vi "Load Plugin Management.vi"(11 "CIFPluginManager in":refnum<class "CIFPluginManager.lvclass">) -> (0 "error out":errorcluster)   [LabVIEW 2021, in "CIFPluginManager.lvclass"]
uses:
  CIFPluginManager.lvclass
  CIFPluginManager.lvclass/CIFPluginManager.ctl
  gRPC/CIF_Manager_server/RPC Service/Manager/Manager.lvclass
  C:/Program Files/National Instruments/LabVIEW 2021/vi.lib/gRPC/LabVIEW gRPC Servicer/ServiceBase/ServiceBase.lvclass
  gRPC/CIF_Manager_server/RPC Service/Manager/Manager.lvclass/Manager.ctl
  CIFCore/Common/Typedef/Errors.ctl
  <vilib>/Utility/miscctls.llb/LVMapReplaceAction.ctl
  <vilib>/CIF Foundation/CIF Utilities/Errors/Append Error Location.vi
  <vilib>/CIF Foundation/CIF Utilities/Time/System Time/LabVIEW Time to TAI Time.vi
  <vilib>/string/Create NI GUID.vi
  CIFUtilities/CIFLogs/CIFLogs.lvlib
  CIFCore/Common/CIFCoreCommon.lvlib
  CIFCore/Grpc/CIFCoreWrapper/CIFCoreWrapper.lvlib
  <vilib>/CIF Foundation/CIF Utilities/Time/Time_CIF_U.lvlib
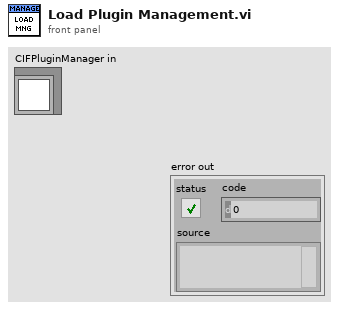
[diagram p1: front panel]
types:
  T1 = typedef "CIF_Manager_server.lvlib/Manager.lvclass/Server gRPC UEs.ctl" = cluster{"Manager LoadPlugin gRPC UE":refnum<user-event>, "Manager RegisterPlugin gRPC UE":refnum<user-event>, "Manager UnregisterPlugin gRPC UE":refnum<user-event>, "Manager QueryPluginTypes gRPC UE":refnum<user-event>, "Manager AbortPlugin gRPC UE":refnum<user-event>, "Manager UnloadAllPlugins gRPC UE":refnum<user-event>, "Manager Destroy gRPC UE":refnum<user-event>, "Manager Ping gRPC UE":refnum<user-event>, "Manager QueryErrors gRPC UE":refnum<user-event>, "Manager QueryConfig gRPC UE":refnum<user-event>, "Manager QueryInfo gRPC UE":refnum<user-event>, "Manager ResetErrorIndex gRPC UE":refnum<user-event>, "Manager ResetConfigIndex gRPC UE":refnum<user-event>, "Manager ResetInfoIndex gRPC UE":refnum<user-event>, "Manager QueryPluginInfo gRPC UE":refnum<user-event>, "Manager QueryPlugin gRPC UE":refnum<user-event>, "Manager QuerySystemStatus gRPC UE":refnum<user-event>, "Manager UpdateClock gRPC UE":refnum<user-event>, "Manager CreateOrch gRPC UE":refnum<user-event>, "Manager QueryClockStatus gRPC UE":refnum<user-event>, "Manager QueryAllChannels gRPC UE":refnum<user-event>}
  T2 = typedef "CIFCoreCommon.lvlib/Errors.ctl" = enum16{"Invalid Clock ID", "Long Sleep", "gRPC Server Not Found", "Config Parse", "Timestamp Wrap", "Delayed Execution", "Duplicate Channel", "Missing Channel", "Incorrect Type", "Flatten Error", "Unflatten Data", "Unique Name", "Plugin Not Found", "Plugin Type Not Found", "Plugin Version Not Found", "Manager Not Found", "Numerical Issue", "Time Jump", "Clock ID Match", "Channel Length", "Plugin Connection", "gRPC Server Connection", "PPL Name Match", "Build", "Config Log Parse", "Plugin Load", "UI Subpanel Load", "Python Name", "Invalid Name", "Unable to Change Ch Buffer"}
  T3 = typedef "LVMapReplaceAction.ctl" = enum32{"Modify Entry only if found", "Add or Modify Entry", "Delete Entry"}
  T4 = typedef "CIFPluginManager.lvclass/Plugin Management Data Map.ctl" = map{string, T5}
  T5 = typedef "CIFPluginManager.lvclass/Plugin Management Data.ctl" = cluster{"vi reference":refnum<vi>, "gRPC ID":T6, "Plugin Type":string, "Unique Name":string, "gRPC Port":i32, "Version":T7, "Load Timestamp":i64, "Unload Timestamp":i64, "Unloading":bool, "Ready for removal":bool, "status":T8}
  T6 = typedef "grpc-lvsupport-release.lvlib/grpcId.ctl" = u64
  T7 = typedef "CIFCoreCommon.lvlib/Version.ctl" = cluster{"Major":i32, "Minor":i32, "Fix":i32, "Build":i32}
  T8 = typedef "CIF_Manager_server.lvlib/cif_plugincore_StatusData.ctl" = cluster{"state":T9, "timing_statistics":T10, "fifo_statistics":T12, "error":T13, "monitor_doubles":T14, "monitor_u64s":T15, "monitor_i64s":T16}
  T9 = typedef "CIF_Manager_server.lvlib/cif_plugincore_StatusData_State.ctl" = enum32{"NULL", "CREATING", "LISTENING", "RUNNING", "CLEANINGUP", "DESTROYING"}
  T10 = typedef "CIF_Manager_server.lvlib/cif_plugincore_TimingStatistics.ctl" = cluster{"period":T11, "wake_error":T11, "execute":T11, "housekeep":T11, "idle":T11, "cleanup":T11, "custom_1":T11, "custom_2":T11}
  T11 = typedef "CIF_Manager_server.lvlib/cif_common_TimingStats.ctl" = cluster{"max":i64, "min":i64, "avg":dbl}
  T12 = typedef "CIF_Manager_server.lvlib/cif_plugincore_FifoStatistics.ctl" = cluster{"from_t0":T11, "from_previous_plugin":T11, "output_error":T11}
  T13 = typedef "CIF_Manager_server.lvlib/cif_plugincore_Error.ctl" = cluster{"status":bool, "code":i32}
  T14 = typedef "CIF_Manager_server.lvlib/cif_plugincore_MonitorDoubles.ctl" = cluster{"double_1":dbl, "double_2":dbl, "double_3":dbl, "double_4":dbl}
  T15 = typedef "CIF_Manager_server.lvlib/cif_plugincore_MonitorU64.ctl" = cluster{"u64_1":u64, "u64_2":u64, "u64_3":u64, "u64_4":u64}
  T16 = typedef "CIF_Manager_server.lvlib/cif_plugincore_MonitorI64.ctl" = cluster{"i64_1":i64, "i64_2":i64, "i64_3":i64, "i64_4":i64}
  T17 = typedef "CIF_Manager_server.lvlib/cif_manager_PluginConfig.ctl" = cluster{"plugin_type":string, "plugin_name":string, "version":string}
  T18 = typedef "CIFPluginManager.lvclass/Discovered Plugin.ctl" = cluster{"Filename":string, "Plugin Type":string, "Qualified name":string, "Version":T7, "Plugin Metadata":T19}
  T19 = typedef "CIFPluginManager.lvclass/Plugin Metadata.ctl" = cluster{"Description":string, "History":string, "Author":string}
  T20 = typedef "CIF_Manager_client.lvlib/cif_common_Status.ctl" = cluster{"code":i32, "message":string}
  T21 = typedef "CIF_Manager_server.lvlib/cif_manager_PluginName.ctl" = cluster{"plugin_name":string}
  T22 = typedef "Plugin Management Data Map.ctl" = map{string, T5}
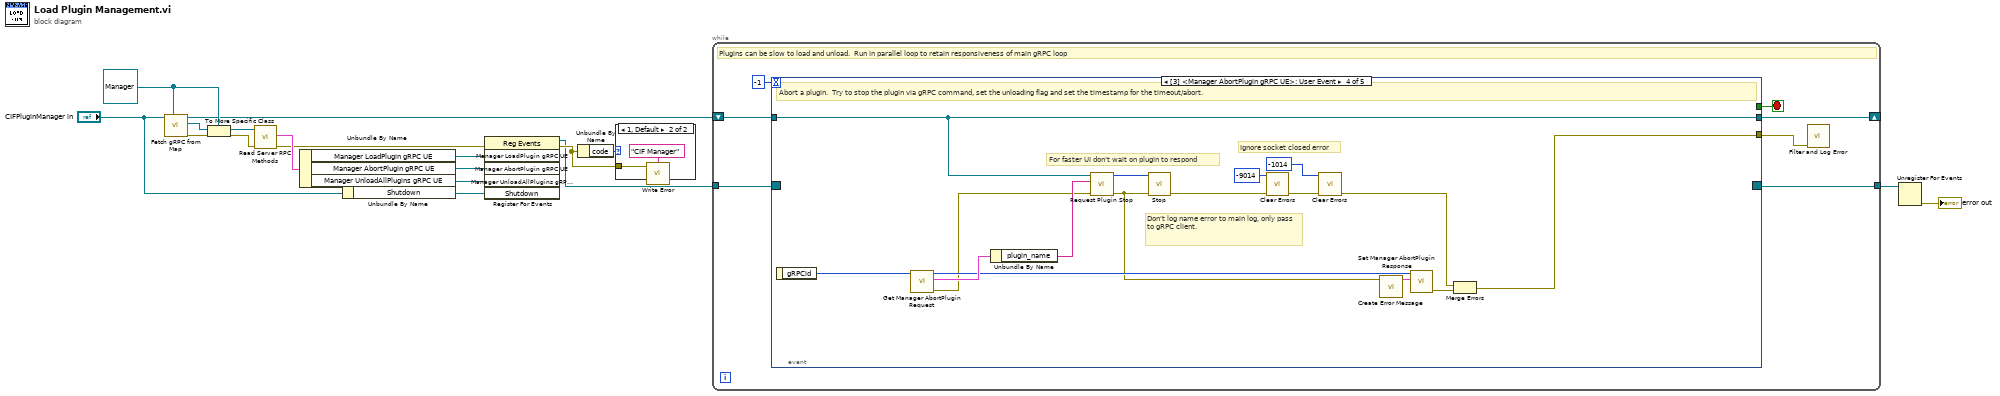
[diagram p0: block diagram]
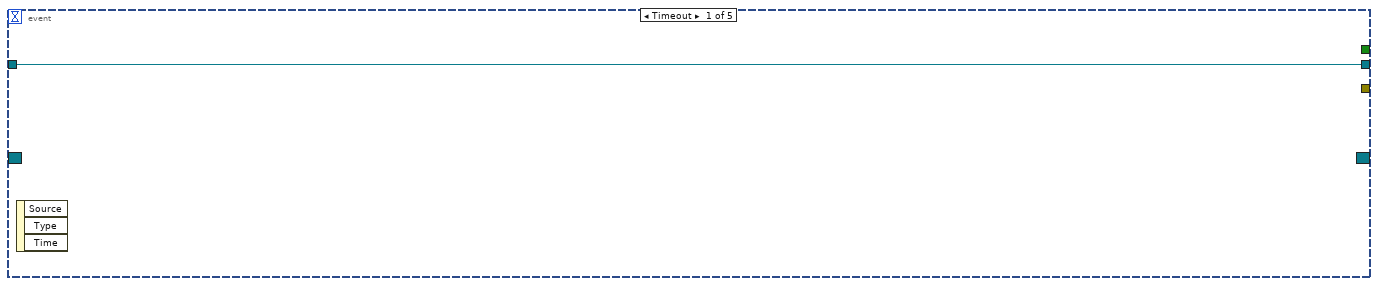
[diagram p3: hidden frame]
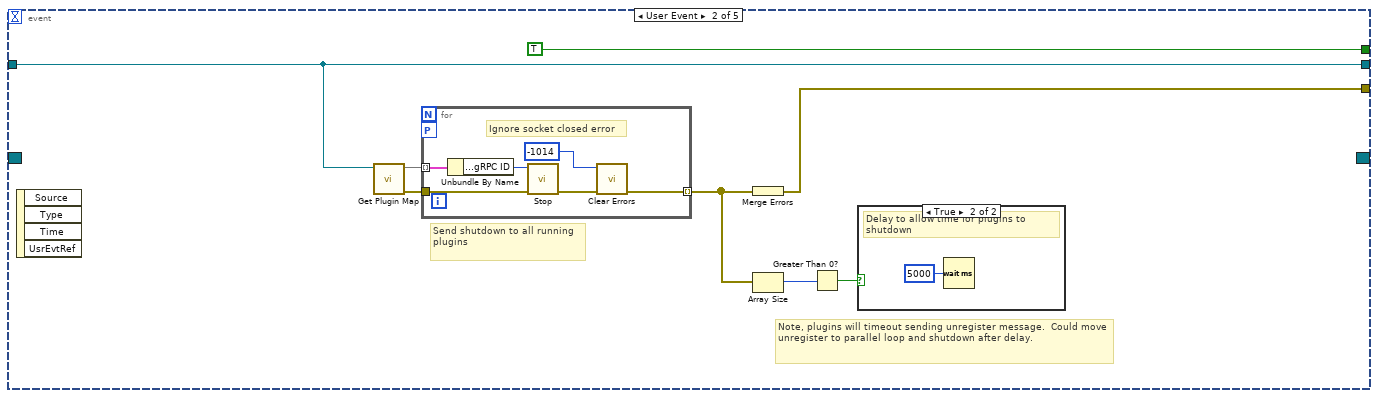
[diagram p4: hidden frame]
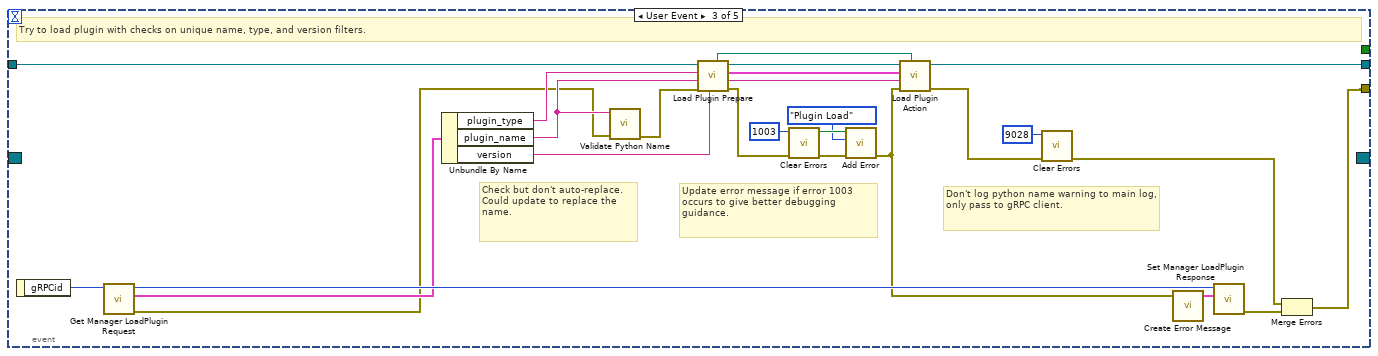
[diagram p6: hidden frame]
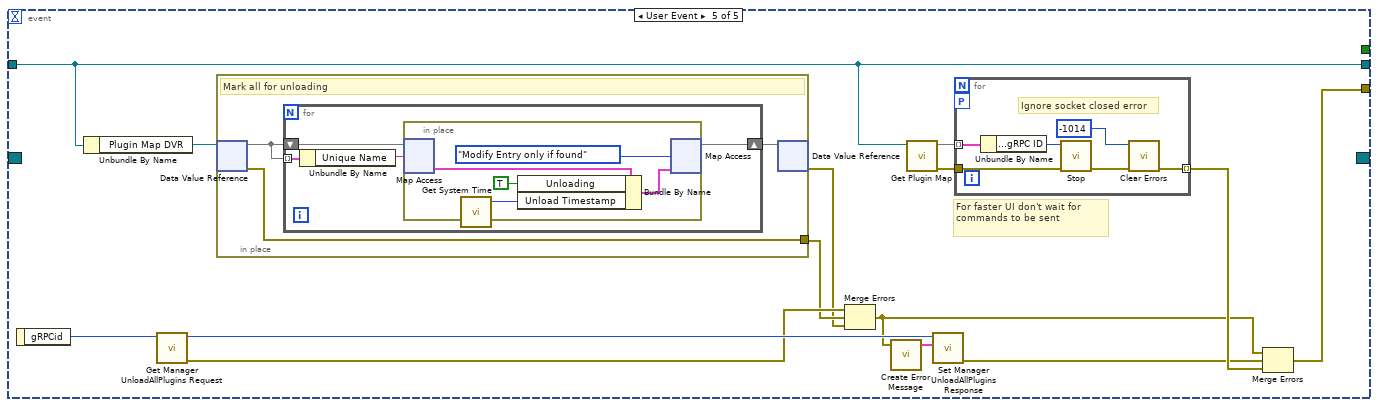
[diagram p7: hidden frame]
diagram:
  w14 = refnum<class "Manager.lvclass"> refnum ("CIF_Manager_server.lvlib:Manager.lvclass")
  n1 = call "Fetch gRPC from Map.vi"("gRPC Server Class type"=w14, "Plugin Manager in"="CIFPluginManager in") -> ("error out"=w13:errorcluster, "gRPC Server Class out"=w15:refnum<class "ServiceBase.lvclass">, "Plugin Manager out"=w7:refnum<class "CIFPluginManager.lvclass">)  [unwired: 7 in]
  n2 = To More Specific Class(target class=w14, reference=w15, error in=w13) -> (specific class reference=w11:refnum<class "Manager.lvclass">, error out=w12:errorcluster)
  n3 = call "Read Server RPC Methods.vi"("error in (no error)"=w12, "SignalGeneratorService in"=w11) -> ("error out"=w5:errorcluster, "Server RPC Methods"=w6:T1)  [unwired: 7 in, 1 out]
  n4 = Unbundle By Name(w6) -> ("Manager LoadPlugin gRPC UE"=w1:refnum<user-event>, "Manager AbortPlugin gRPC UE"=w2:refnum<user-event>, "Manager UnloadAllPlugins gRPC UE"=w3:refnum<user-event>)
  n5 = Unbundle By Name("CIFPluginManager in") -> ("Shutdown"=w4:refnum<user-event>)
  n6 = register-events(error in=w5, w1, w2, w3, w4) -> (reference out=w8:refnum<event-registration>, error out=w9:errorcluster)  [unwired: 1 in]
  n7 = Unbundle By Name(w9) -> ("code"=w16:i32)
  n8 = case shown="1, Default" w16 {
    tunnel: w9 -> [_ w20]
    frame 0 {
      # "-1001 is cancelled by client.  Not an error."
    }
    frame 1, Default {
      n9 = call "Write Error.vi"("error in (no error)"=w20, "Plugin Name"="CIF Manager") -> ()  [unwired: 2 in, 1 out]
    }
  }
  n10 = while {
    tunnel: w8 -> [w21]
    shift-right: [w23] -> _
    shift-left: w7 -> [w27]
    tunnel: [w24] -> w17
    stop <- w25 stop-if-true
    # "Plugins can be slow to load and unload.  Run in parallel loop to retain responsiveness of main gRPC loop"
    n11 = event shown="[3] <Manager AbortPlugin gRPC UE>: User Event" {
      selector: w21 -> [_ _ _ _ _]
      dyn-events: [_ _ _ _ _] -> w24
      timeout: -1 -> [_ _ _ _ _]
      tunnel: w27 -> [w28 w34 w49 w77 w92]
      tunnel: [w28 w34 w51 w77 w92] -> w23
      tunnel: [_ TRUE _ _ _] -> w25
      tunnel: [_ w33 w50 w79 w89] -> w22
      event Timeout {
        n12 = event-data() -> ()  [unwired: 1 in, 3 out]
      }
      event User Event {
        # "Note, plugins will timeout sending unregister message.  Could move unregister to parallel loop and shutdown after delay."
        # "Send shutdown to all running plugins"
        n13 = event-data() -> ()  [unwired: 1 in, 4 out]
        n14 = call "Get Plugin Map.vi"("CIFPluginManager in"=w34) -> ("error out"=w35:errorcluster, "Plugin Map"=w32:T4)  [unwired: 9 in]
        n15 = for {
          tunnel: w35 -> [w41]
          tunnel: w32 -> [w42] mode=indexing
          workers-P: _ -> [_]
          tunnel: [w38] -> w31 mode=indexing
          # "Ignore socket closed error"
          n16 = Unbundle By Name(w42) -> ("Plugin Management Data.gRPC ID"=w43:T6)
          n17 = call "Stop.vi"("error in"=w41, "gRPC ID"=w43) -> ("error out"=w39:errorcluster)  [unwired: 8 in, 1 out]
          n18 = call <vilib>:"Clear Errors.vi"("error in (no error)"=w39, "specific error code to clear (0: all)"=-1014) -> ("error out"=w38:errorcluster)  [unwired: 4 in, 1 out]
        }
        n19 = Merge Errors(w31) -> (w33:errorcluster)
        n20 = Array Size(array=w31) -> (size(s)=w30:i32)
        n21 = Greater Than 0?(x=w30) -> (x > 0?=w29:bool)
        n22 = case shown="True" w29 {
          frame False {
          }
          frame True {
            # "Delay to allow time for plugins to shutdown"
            n23 = Wait (ms)(milliseconds to wait=u32 5000) -> ()  [unwired: 1 out]
          }
        }
      }
      event User Event {
        # "Don't log python name warning to main log, only pass to gRPC client."
        # "Check but don't auto-replace.  Could update to replace the name."
        # "Update error message if error 1003 occurs to give better debugging guidance."
        # "Try to load plugin with checks on unique name, type, and version filters."
        n24 = event-data() -> ("gRPCid"=w48:T6)  [unwired: 1 in]
        n25 = call "Get Manager LoadPlugin Request.vi"("gRPCid"=w48) -> ("error out"=w57:errorcluster, "Message Data"=w66:T17, "gRPCid out"=w69:T6)  [unwired: 8 in]
        n26 = Unbundle By Name(w66) -> ("plugin_type"=w65:string, "plugin_name"=w58:string, "version"=w64:string)
        n27 = call "Validate Python Name.vi"("error in (no error)"=w57, "Name In"=w58) -> ("error out"=w59:errorcluster)  [unwired: 8 in, 1 out]
        n28 = call "Load Plugin Prepare.vi"("Version String"=w64, "error in (no error)"=w59, "Unique Name"=w58, "Plugin Type"=w65, "Launcher in"=w49) -> ("error out"=w56:errorcluster, "Unique Name (dup)"=w54:string, "Matching Plugin"=w53:T18, "Launcher (dup)"=w55:refnum<class "CIFPluginManager.lvclass">, "path"=w52:path)  [unwired: 2 in]
        n29 = call <vilib>:"Clear Errors.vi"("error in (no error)"=w56, "specific error code to clear (0: all)"=1003) -> ("error out"=w63:errorcluster, "specific error cleared?"=w61:bool)  [unwired: 4 in]
        n30 = call "Add Error.vi"("error in (no error)"=w63, "Error"=Errors."Plugin Load", "Insert Error"=w61) -> ("error out"=w45:errorcluster)  [unwired: 8 in]
        n31 = call "Load Plugin Action.vi"("plugin path"=w52, "error in (no error)"=w45, "Unique Name"=w54, "Plugin"=w53, "Launcher in"=w55) -> ("error out"=w44:errorcluster, "Launcher out"=w51:refnum<class "CIFPluginManager.lvclass">)  [unwired: 5 in]
        n32 = call <vilib>:"Clear Errors.vi"("error in (no error)"=w44, "specific error code to clear (0: all)"=9028) -> ("error out"=w46:errorcluster)  [unwired: 4 in, 1 out]
        n33 = call "Create Error Message.vi"("error in (no error)"=w45) -> ("Error Message"=w68:T20)  [unwired: 3 in]
        n34 = call "Set Manager LoadPlugin Response.vi"("Message Data"=w68, "gRPCid in"=w69) -> ("error out"=w67:errorcluster)  [unwired: 9 in]
        n35 = Merge Errors(w46, w67) -> (w50:errorcluster)
      }
      event User Event {
        # "Ignore socket closed error"
        # "Don't log name error to main log, only pass to gRPC client."
        # "For faster UI don't wait on plugin to respond"
        # "Abort a plugin.  Try to stop the plugin via gRPC command, set the unloading flag and set the timestamp for the timeout/abort."
        n36 = event-data() -> ("gRPCid"=w80:T6)  [unwired: 1 in]
        n37 = call "Get Manager AbortPlugin Request.vi"("gRPCid"=w80) -> ("error out"=w78:errorcluster, "Message Data"=w83:T21, "gRPCid out"=w81:T6)  [unwired: 8 in]
        n38 = Unbundle By Name(w83) -> ("plugin_name"=w85:string)
        n39 = call "Request Plugin Stop.vi"("error in (no error)"=w78, "Unique Name"=w85, "CIFPluginManager in"=w77) -> ("error out"=w75:errorcluster, "gRPC ID"=w76:T6)  [unwired: 7 in]
        n40 = call "Stop.vi"("error in"=w75, "gRPC ID"=w76) -> ("error out"=w73:errorcluster)  [unwired: 8 in, 1 out]
        n41 = call <vilib>:"Clear Errors.vi"("error in (no error)"=w73, "specific error code to clear (0: all)"=-9014) -> ("error out"=w71:errorcluster)  [unwired: 4 in, 1 out]
        n42 = call <vilib>:"Clear Errors.vi"("error in (no error)"=w71, "specific error code to clear (0: all)"=-1014) -> ("error out"=w70:errorcluster)  [unwired: 4 in, 1 out]
        n43 = call "Create Error Message.vi"("error in (no error)"=w75) -> ("Error Message"=w84:T20)  [unwired: 3 in]
        n44 = call "Set Manager AbortPlugin Response.vi"("Message Data"=w84, "gRPCid in"=w81) -> ("error out"=w82:errorcluster)  [unwired: 9 in]
        n45 = Merge Errors(w70, w82) -> (w79:errorcluster)
      }
      event User Event {
        # "For faster UI don't wait for commands to be sent"
        n46 = event-data() -> ("gRPCid"=w98:T6)  [unwired: 1 in]
        n47 = Unbundle By Name(w92) -> ("Plugin Map DVR"=w99:refnum<data-value>)
        n48 = call "Get Manager UnloadAllPlugins Request.vi"("gRPCid"=w98) -> ("error out"=w95:errorcluster, "gRPCid out"=w96:T6)  [unwired: 8 in, 1 out]
        n49 = in-place {
          in-place-border: [w106] -> w94
          # "Mark all for unloading"
          n50 = in-place-dvr #1(w99) -> (w108:T22, w106:errorcluster)
          n51 = for {
            tunnel: w108 -> [w110] mode=indexing
            shift-right: [w111] -> w107
            shift-left: w108 -> [w112]
            n52 = Unbundle By Name(w110) -> ("Unique Name"=w109:string)
            n53 = in-place {
              n54 = in-place-map #2(w112, w109) -> (w114:T5)  [unwired: 1 in, 1 out]
              n55 = call <vilib>:"Get System Time.vi"() -> ("Time (ns)"=w115:i64)  [unwired: 5 in]
              n56 = Bundle By Name(cluster=w114, "Unloading"=TRUE, "Unload Timestamp"=w115) -> (w113:T5)
              n57 = in-place-map #2(w113, LVMapReplaceAction."Modify Entry only if found" ("action")) -> (w111:T22)  [unwired: 2 out]
            }
          }
          n58 = in-place-dvr #1(w107) -> (w93:errorcluster)  [unwired: 1 out]
        }
        n59 = Merge Errors(w95, w94, w93) -> (w87:errorcluster)
        n60 = call "Create Error Message.vi"("error in (no error)"=w87) -> ("Error Message"=w97:T20)  [unwired: 3 in]
        n61 = call "Get Plugin Map.vi"("CIFPluginManager in"=w92) -> ("error out"=w90:errorcluster, "Plugin Map"=w91:T4)  [unwired: 9 in]
        n62 = call "Set Manager UnloadAllPlugins Response.vi"("Message Data"=w97, "gRPCid in"=w96) -> ("error out"=w86:errorcluster)  [unwired: 9 in]
        n63 = for {
          tunnel: w90 -> [w103]
          tunnel: w91 -> [w104] mode=indexing
          workers-P: _ -> [_]
          tunnel: [w101] -> w88 mode=indexing
          # "Ignore socket closed error"
          n64 = Unbundle By Name(w104) -> ("Plugin Management Data.gRPC ID"=w105:T6)
          n65 = call "Stop.vi"("error in"=w103, "gRPC ID"=w105) -> ("error out"=w102:errorcluster)  [unwired: 8 in, 1 out]
          n66 = call <vilib>:"Clear Errors.vi"("error in (no error)"=w102, "specific error code to clear (0: all)"=-1014) -> ("error out"=w101:errorcluster)  [unwired: 4 in, 1 out]
        }
        n67 = Merge Errors(w87, w86, w88) -> (w89:errorcluster)
      }
    }
    n68 = call "Filter and Log Error.vi"("error In"=w22) -> ()  [unwired: 11 in]
  }
  n69 = Unregister For Events(event registration refnum=w17) -> (error out=→"error out":errorcluster)  [unwired: 1 in]
